vi "Initialize Input Gain.vi"(8 "error in (no error)":errorcluster, 11 "Instrument.Lockin":refnum<class "Instrument.Lockin.lvclass">) -> (0 "error out":errorcluster, 2 "Input Gain":cluster{string, "Gain":dbl}[](array[cluster]), 3 "Instrument.Lockin out":refnum<class "Instrument.Lockin.lvclass">)   [LabVIEW 2019, in "Instrument.Lockin.lvclass"]
uses:
  Instrument.Lockin.lvclass
  Instrument.Lockin.lvclass/Instrument.Lockin.ctl
  Instrument.DAQ/Instrument.DAQ.lvclass
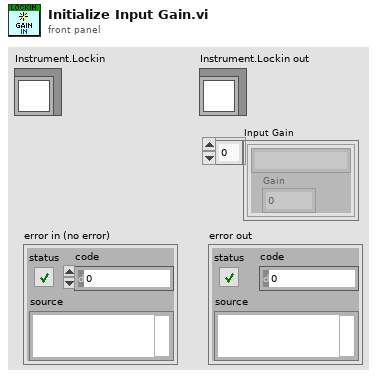
[diagram p1: front panel]
types:
  T1 = typedef "Instrument.DAQ.lvclass/DAQ.Config.AI--Cluster--Array.ctl" = T2[]
  T2 = typedef "Instrument.DAQ.lvclass/DAQ.Config.AI--Cluster.ctl" = cluster{"Channels":tag, "Coupling":T3, "Range":T4, "input terminal configuration":i32, "Type":T5}
  T3 = typedef "Instrument.DAQ.lvclass/DAQ.Config.AI.Coupling--enum.ctl" = u16
  T4 = typedef "Instrument.DAQ.lvclass/DAQ.Config.AI.Range--enum.ctl" = enum16{"±0.316", "±1.00", "±3.16", "±10.0", "±31.6", "±42.4"}
  T5 = typedef "Instrument.DAQ.lvclass/DAQ.Type--enum.ctl" = enum16{"None", "USB 4431", "PXI 446x"}
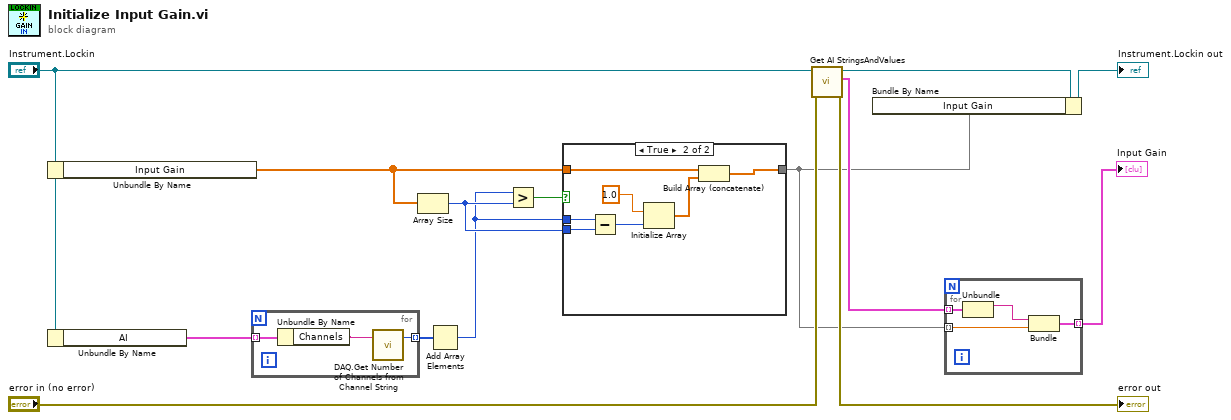
[diagram p0: block diagram]
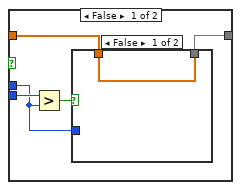
[diagram p2: hidden frame]
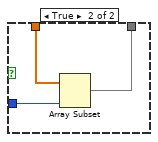
[diagram p3: hidden frame]
diagram:
  n1 = Unbundle By Name("Instrument.Lockin") -> ("Input Gain"=w10:dbl[])
  n2 = Unbundle By Name("Instrument.Lockin") -> ("AI"=w14:T1)
  n3 = for {
    tunnel: w14 -> [w17] mode=indexing
    tunnel: [w15] -> w12 mode=indexing
    n4 = Unbundle By Name(w17) -> ("Channels"=w16:tag)
    n5 = call "DAQ.Get Number of Channels from Channel String.vi"("Channels String"=w16) -> ("# channels"=w15:i32)  [unwired: 2 in]
  }
  n6 = Array Size(array=w10) -> (size(s)=w11:i32)
  n7 = Add Array Elements(numeric array=w12) -> (sum=w9:i32)
  n8 = Greater?(x=w9, y=w11) -> (0:w13:bool)
  n9 = case shown="True" w13 {
    tunnel: [w19 w27] -> w2
    tunnel: w10 -> [w20 w29]
    tunnel: w9 -> [w18 w32]
    tunnel: w11 -> [w22 w31]
    frame False {
      n10 = Greater?(x=w22, y=w18) -> (0:w21:bool)
      n11 = case shown="False" w21 {
        tunnel: w20 -> [w23 w26]
        tunnel: [w23 w24] -> w19
        tunnel: w18 -> [_ w25]
        frame False {
        }
        frame True {
          n12 = Array Subset(array=w26, length=w25) -> (w24:dbl[])  [unwired: 1 in]
        }
      }
    }
    frame True {
      n13 = Subtract(x=w32, y=w31) -> (x-y=w30:i32)
      n14 = Initialize Array(1.0, w30) -> (w28:dbl[])
      n15 = Build Array (concatenate)(w29, w28) -> (w27:dbl[])
    }
  }
  n16 = call "Get AI StringsAndValues.vi"("error in (no error)"="error in (no error)", "Instrument.Lockin in"="Instrument.Lockin") -> ("error out"=→"error out":errorcluster, "AI StringsAndValues"=w7:cluster{string, i32}[], "Instrument.Lockin out"=w5:refnum<class "Instrument.Lockin.lvclass">)  [unwired: 7 in]
  n17 = Bundle By Name(cluster=w5, "Input Gain"=w2) -> (→"Instrument.Lockin out":refnum<class "Instrument.Lockin.lvclass">)
  n18 = for {
    tunnel: [w37] -> w1 mode=indexing
    tunnel: w2 -> [w36] mode=indexing
    tunnel: w7 -> [w35] mode=indexing
    n19 = Unbundle(w35) -> (w34:string)  [unwired: 1 out]
    n20 = Bundle(w34, "Gain"=w36) -> (w37:cluster{string, "Gain":dbl})  [unwired: 1 in]
  }
  "Input Gain" <- w1
